vi "Staging_CapSideView.vi"() -> ()   [LabVIEW 2020]
uses:
  Shared/GUI_Template/GUI_master/tcp new data cluster.ctl
  Shared/GUI_Template/GUI_master/tcp_new_data_event.ctl
  Device Driver/FilterWheels/posTypDef.ctl
panel:
  out "Max Counts":dbl(slide) scale=0.0..256.0
  in  "triggerdelay::1":dbl caption="trigger delay" min=0.0 max=0.09 format="%.6g"
  in  "save::1":bool caption="Save"
  in  "trigger::1":bool caption="Trigger"
  in  "pos.Channel0::3":T1=enum."3" caption="filter wheel"
  in  "GUIdevice 3":string="StagingRS232FilterWheels"
  in  "DigitalOutput.Channel 0::2":bool caption="light"
  in  "GUIdevice 2":string="Staging_USB6210_1"
  out "image::1":T2(plugin-control) caption="Image"
  in  "stop":bool
  in  "exposure::1":dbl caption="exposure" min=0.0001 max=1.0
  in  "GUIdevice 1":string="StagingSideView"
  out "tcp data event":T3
  out "error IO 2":errorcluster
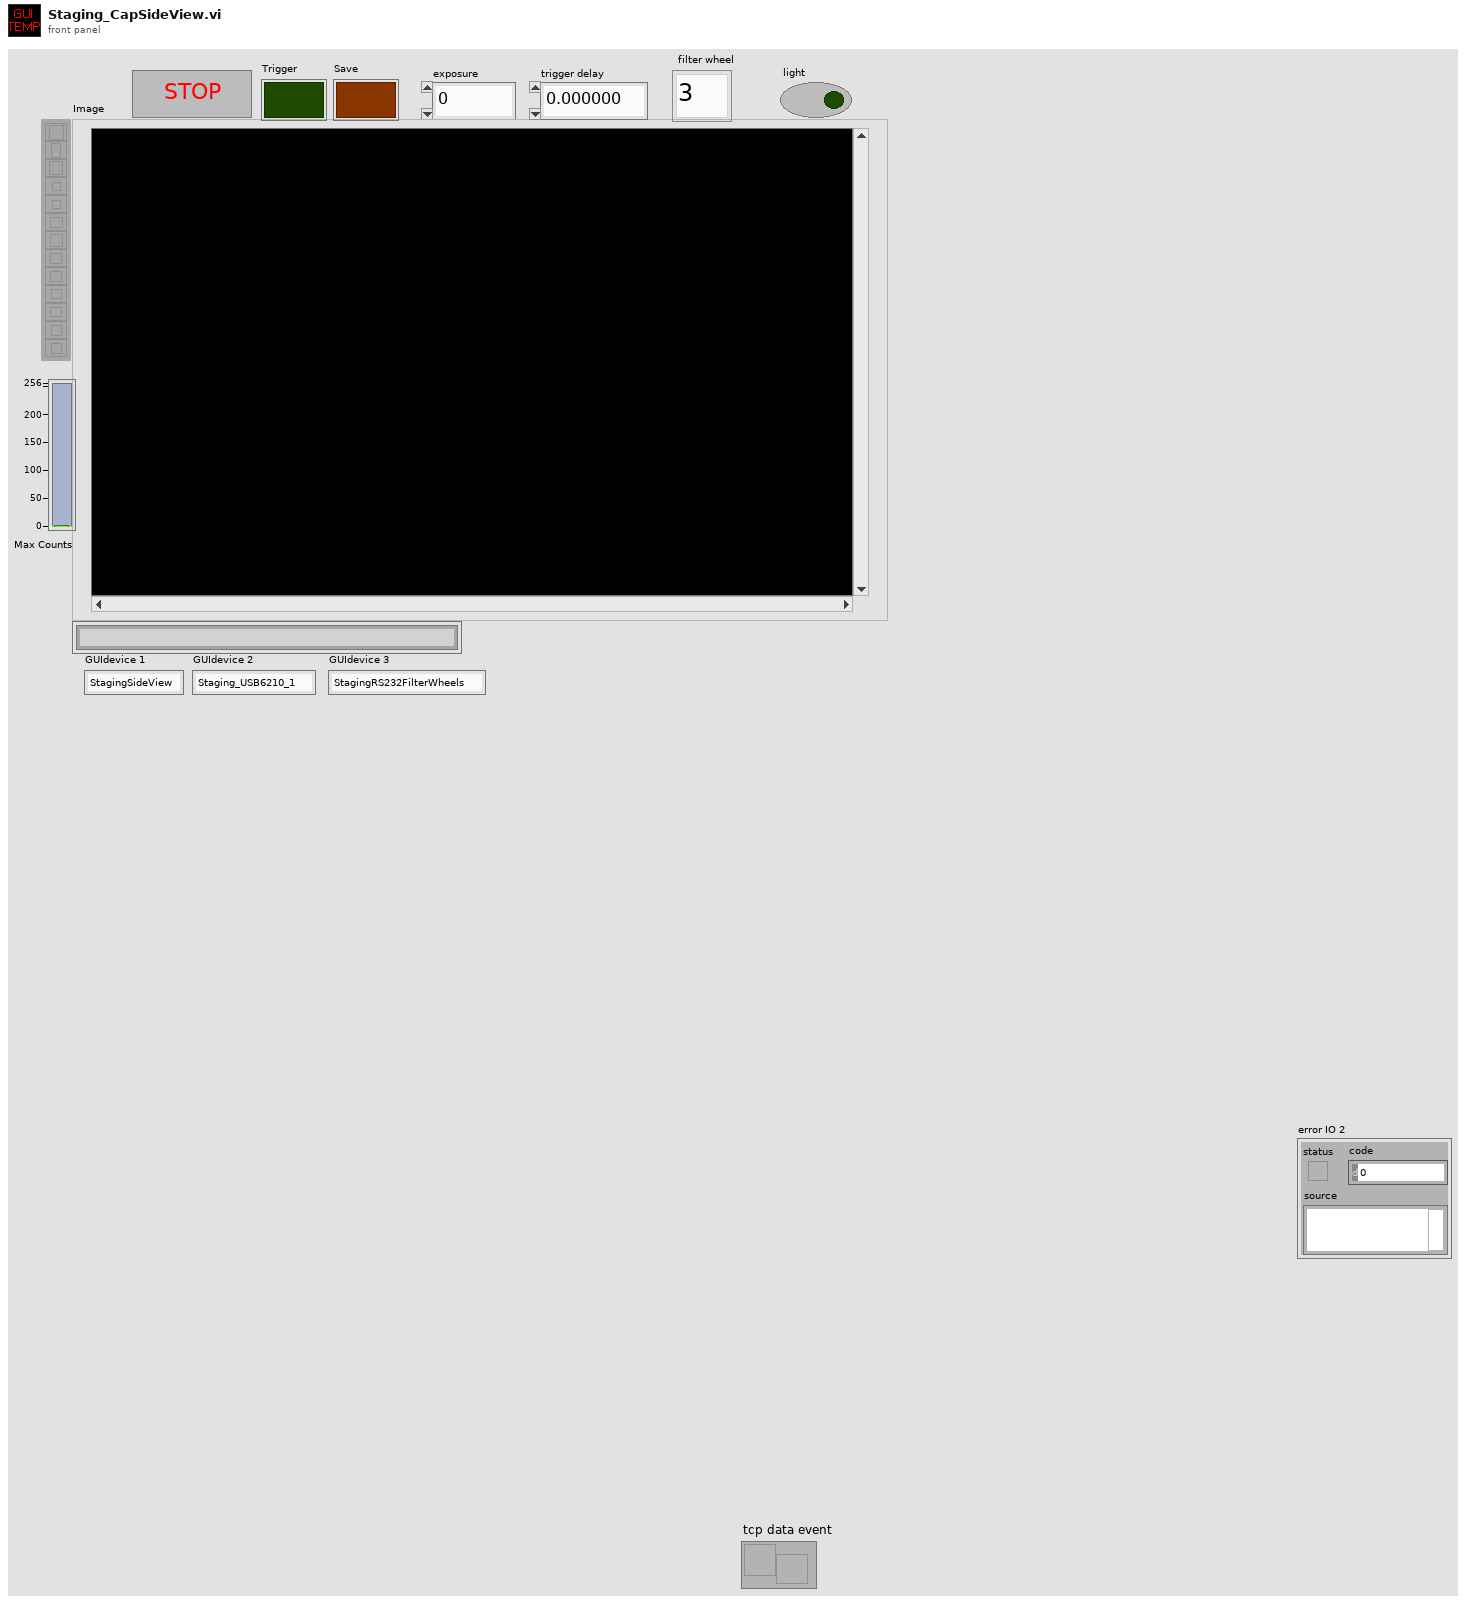
[diagram p1: front panel]
types:
  T1 = typedef "posTypDef.ctl" = enum16{"1", "2", "3", "4", "5", "6"}
  T2 = typedef "IMAQ Image.ctl" = refnum<image>
  T3 = typedef "tcp_new_data_event.ctl" = refnum<user-event>
  T4 = typedef "tcp new data cluster.ctl" = cluster{"EventEnum":enum16{"new data", "connection status update"}, "Device name":string}
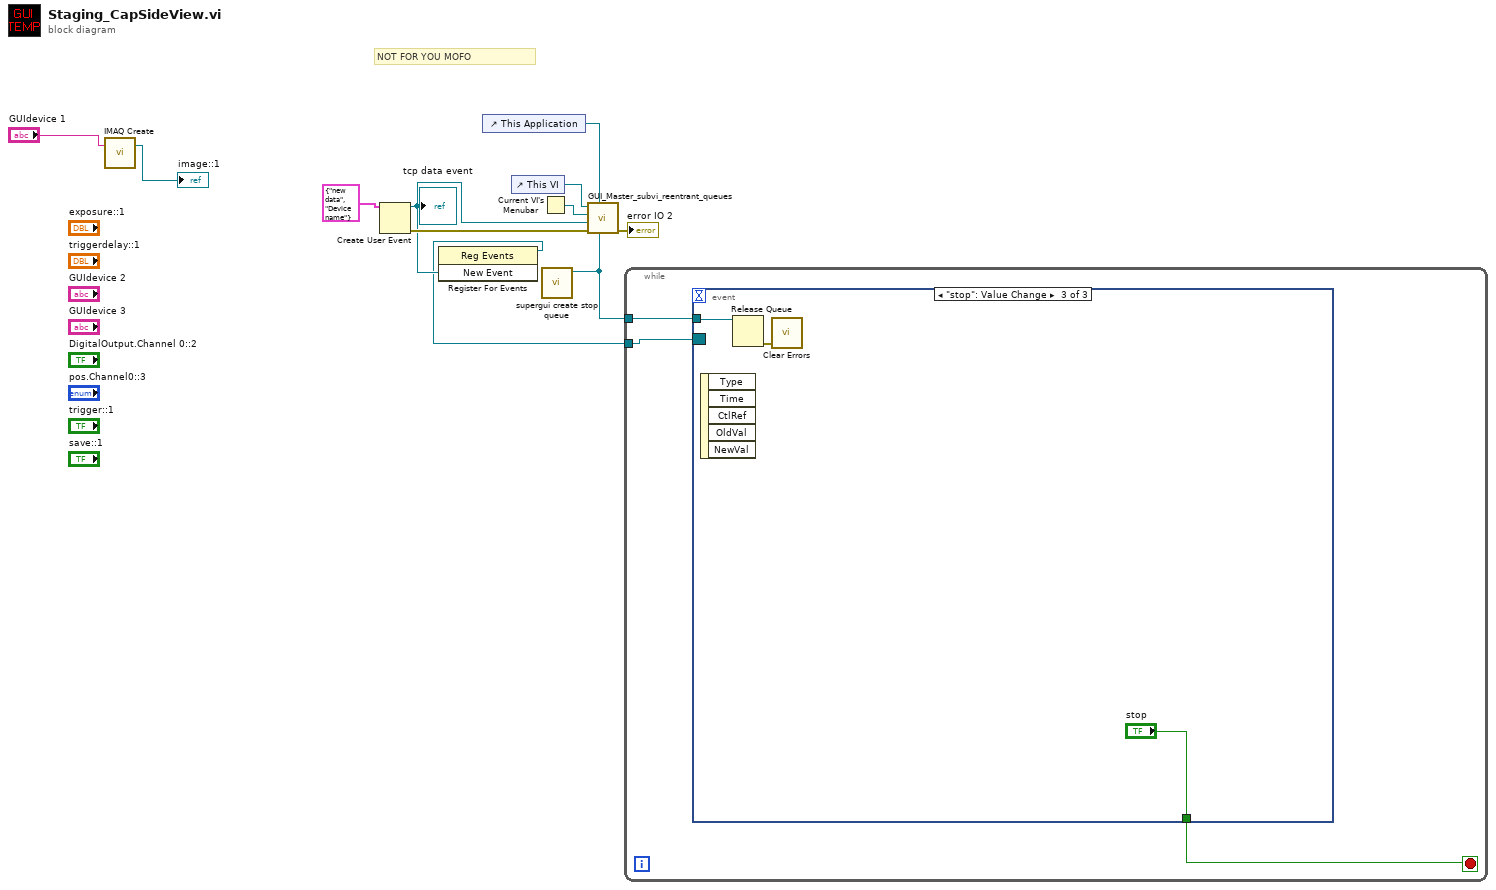
[diagram p0: block diagram]
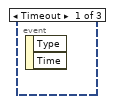
[diagram p2: hidden frame]
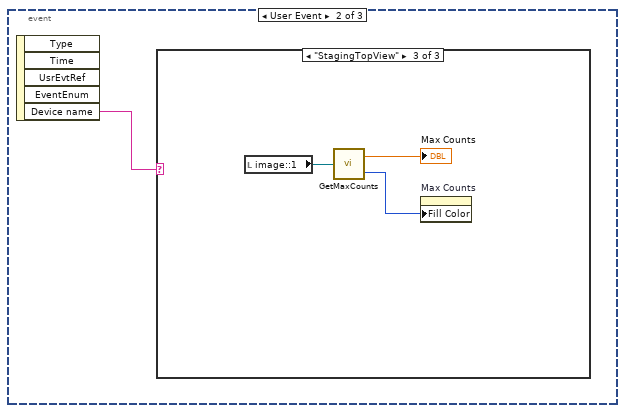
[diagram p3: hidden frame]
diagram:
  # "NOT FOR YOU MOFO"
  n1 = call "IMAQ Create"("Image Name"="GUIdevice 1") -> ("New Image"=→"image::1":T2)  [unwired: 4 in, 1 out]
  n2 = Create User Event(user event datatype=T4 {"EventEnum"=enum."new data", "Device name"="Device name"} ("New Event")) -> (user event=w6:refnum<user-event>, error out=w7:errorcluster)  [unwired: 1 in]
  "tcp data event" <- w6
  n3 = register-events(w6) -> (reference out=w4:refnum<event-registration>)  [unwired: 2 in, 1 out]
  n4 = control-ref of="This Application"() -> (w5:refnum<vi>)
  n5 = control-ref of="This VI"() -> (w10:refnum<vi>)
  n6 = Current VI's Menubar() -> (w9:refnum<k9>)
  n7 = call "supergui create stop queue.vi"() -> ("STOP Queue out"=w1:refnum<queue>)  [unwired: 11 in]
  n8 = call "GUI_Master_subvi_reentrant_queues.vi"("STOP Queue in"=w1, "This Application"=w5, "error in (no error)"=w7, "tcp data event"=w6, "Caller menu reference"=w9, "Caller VI ref"=w10) -> ("error out"=→"error IO 2":errorcluster)  [unwired: 5 in]
  n9 = while {
    tunnel: w4 -> [w14]
    tunnel: w1 -> [w12]
    stop <- w13 stop-if-true
    n10 = event shown="[2] \"stop\": Value Change" {
      selector: w14 -> [_ _ _]
      dyn-events: _ -> [_ _ _]
      timeout: _ -> [_ _ _]
      tunnel: [_ _ "stop"] -> w13
      tunnel: w12 -> [_ _ w20]
      event Timeout {
        n11 = event-data() -> ()  [unwired: 1 in, 2 out]
      }
      event User Event {
        n12 = event-data() -> ("Device name"=w15:string)  [unwired: 1 in, 4 out]
        n13 = case shown="\"StagingTopView\"" w15 {
          frame "Staging_USB6210_1" {
          }
          frame "StagingRS232FilterWheels", Default {
          }
          frame "StagingTopView" {
            n14 = local read "image::1"() -> (w16:T2)
            n15 = call "GetMaxCounts.vi"("New Image"=w16) -> ("Maximal Value"=→"Max Counts":sgl, "Color"=w17:u32)
            n16 = property on="Max Counts" class="Slide (strict)"("Fill Color"=w17) -> ()  [unwired: 2 in, 2 out]
          }
        }
      }
      event "stop": Value Change {
        n17 = event-data() -> ()  [unwired: 1 in, 5 out]
        n18 = Release Queue(queue=w20) -> (error out=w19:errorcluster)  [unwired: 2 in, 2 out]
        n19 = call <vilib>:"Clear Errors.vi"("error in (no error)"=w19) -> ()  [unwired: 5 in, 2 out]
      }
    }
  }
